vi "Request Token.vi"(5 "Version":string="1.0", 6 "Callback URL":string="oob", 7 "Signature Method":T2=enum."HMAC-SHA1", 8 "error in (no error)":errorcluster, 9 "Consumer Secret":string, 10 "Consumer Key":string, 11 "Request URL":string) -> (0 "error out":errorcluster, 1 "OAuth Credentials (request)":T1={"Signature Method"=enum."HMAC-SHA1", "Version"="", "Client"={"Token"="", "Secret"=""}, "Access"={"Token"="", "Secret"=""}}, 2 "Request Token (duplicate)":string)   [LabVIEW 2011, in "i3-oauth.lvlib"]
doc: "Obtains a request token for the application specified by the <B>Consumer Key</B> and <B>Consumer Secret</B>."
uses:
  i3-oauth.lvlib
  Controls/Signature Method.ctl
  Controls/OAuth Handle.ctl
  Controls/Credentials.ctl
  Controls/HTTP Method.ctl
  <vilib>/httpClient/POSTBuffer.vi
  <vilib>/httpClient/LabVIEWHTTPClient.lvlib
panel:
  out "body":string
  out "headers":string
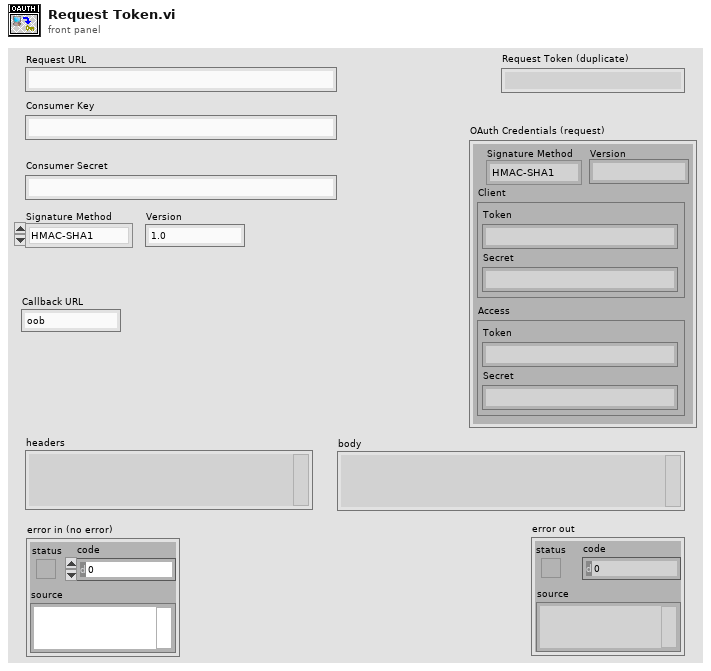
[diagram p1: front panel]
types:
  T1 = typedef "i3-oauth.lvlib/OAuth Handle.ctl" = cluster{"Signature Method":T2, "Version":string, "Client":T3, "Access":T3}
  T2 = typedef "i3-oauth.lvlib/Signature Method.ctl" = enum16{"HMAC-MD5", "HMAC-SHA1", "HMAC-SHA224", "HMAC-SHA256", "HMAC-SHA384", "HMAC-SHA512"}
  T3 = typedef "i3-oauth.lvlib/Credentials.ctl" = cluster{"Token":string, "Secret":string}
  T4 = typedef "i3-oauth.lvlib/HTTP Method.ctl" = enum16{"GET", "POST", "PUT", "DELETE"}
  T5 = typedef "i3-oauth.lvlib/Name-Value Pair.ctl" = cluster{"Name":string, "Value":string}
  T6 = typedef "LabVIEWHTTPClient.lvlib/ClientHandle.ctl" = refnum<k1>
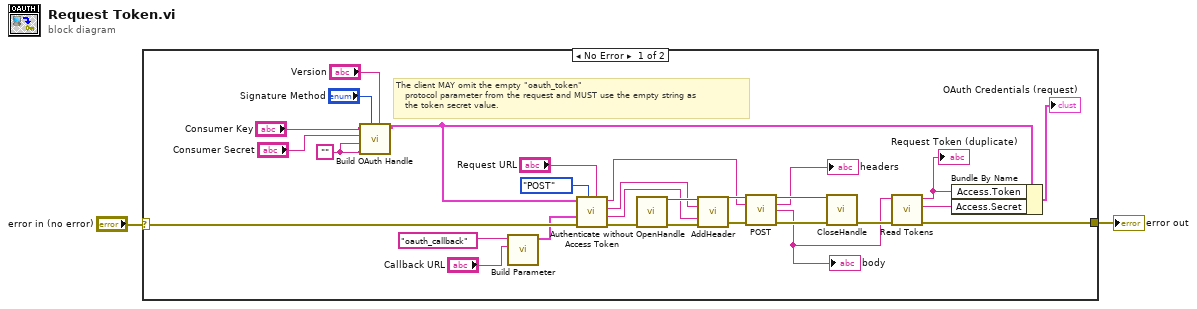
[diagram p0: block diagram]
diagram:
  n1 = case shown="No Error" "error in (no error)" {
    selector: "error in (no error)" -> [w31 w32]
    tunnel: [w23 w32] -> w1
    frame No Error {
      w3 = ""
      # "The client MAY omit the empty \"oauth_token\"\n   protocol parameter from the request and MUST use the empty string as\n   the token secret value."
      n2 = call "Build OAuth Handle.vi"("Version (1.0)"="Version", "Signature Method (HMAC-SHA1)"="Signature Method", "Access Secret"=w3, "Access Token"=w3, "Client Secret"="Consumer Secret", "Client Token"="Consumer Key") -> ("OAuth Handle"=w8:T1)  [unwired: 5 in]
      n3 = call "Build Parameter.vi"("Value"="Callback URL", "Key"="oauth_callback") -> ("Parameter Array"=w15:T5[])  [unwired: 9 in]
      n4 = call "Authenticate without Access Token.vi"("Base URL"="Request URL", "HTTP Method"=HTTP_Method."POST", "error in (no error)"=w31, "Header Parameters"=w15, "OAuth Handle"=w8) -> ("error out"=w11:errorcluster, "Header Value"=w13:string, "Header Parameter"=w14:string, "Full URL"=w12:string)  [unwired: 2 in, 1 out]
      n5 = call <vilib>:"OpenHandle.vi"("error in (no error)"=w11) -> ("client handle out"=w30:T6, "error out"=w29:errorcluster)  [unwired: 13 in]
      n6 = call <vilib>:"AddHeader.vi"("client handle"=w30, "header"=w14, "value"=w13, "error in (no error)"=w29) -> ("client handle out"=w27:T6, "error out"=w28:errorcluster)  [unwired: 10 in]
      n7 = call-poly <vilib>:"POST.vi"("client handle"=w27, "url"=w12, "error in (no error)"=w28) -> ("client handle out"=w25:T6, "headers"=→"headers":string, "body"=w21:string, "error out"=w26:errorcluster)  [unwired: 9 in]
      "body" <- w21
      n8 = call <vilib>:"CloseHandle.vi"("client handle"=w25, "error in (no error)"=w26) -> ("error out"=w22:errorcluster)  [unwired: 13 in]
      n9 = call "Read Tokens.vi"("error in (no error)"=w22, "input string"=w21) -> ("error out"=w23:errorcluster, "Token Secret"=w19:string, "Token"=w20:string)  [unwired: 7 in]
      "Request Token (duplicate)" <- w20
      n10 = Bundle By Name(cluster=w8, "Access.Token"=w20, "Access.Secret"=w19) -> (→"OAuth Credentials (request)":T1)
    }
    frame Error {
    }
  }
  "error out" <- w1
